vi "Configure Digital Gen Multitone.vi"(6 "Enable Waveform (T: Enable)":bool=TRUE, 7 "Enable EQ Output Modification (T: Enable)":bool=TRUE, 8 "error in (no error)":errorcluster, 9 "Amplitude (0)":dbl, 10 "Channel (0: chA)":i32(ring) items=["chA", "chB"], 11 "VISA resource name":refnum<visa-resource-name>) -> (0 "error out":errorcluster, 3 "VISA resource name out":refnum<visa-resource-name>)   [LabVIEW 2014, in "Stanford Research SR1.lvlib"]
doc: "Configures the attributes for the Digital Generator Multitone.\n\n<b>NOTE</b>: This VI may not be supported by certain models of the SR1."
uses:
  Stanford Research SR1.lvlib
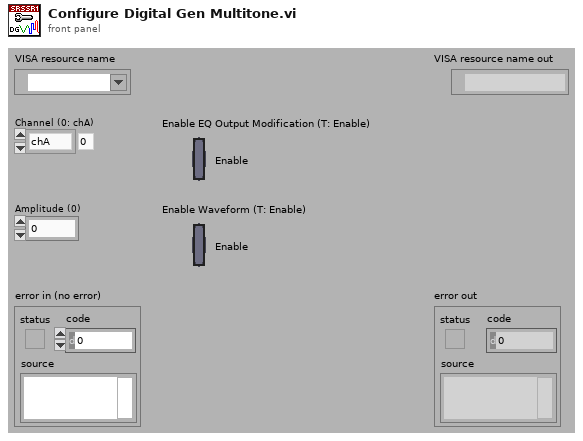
[diagram p1: front panel]
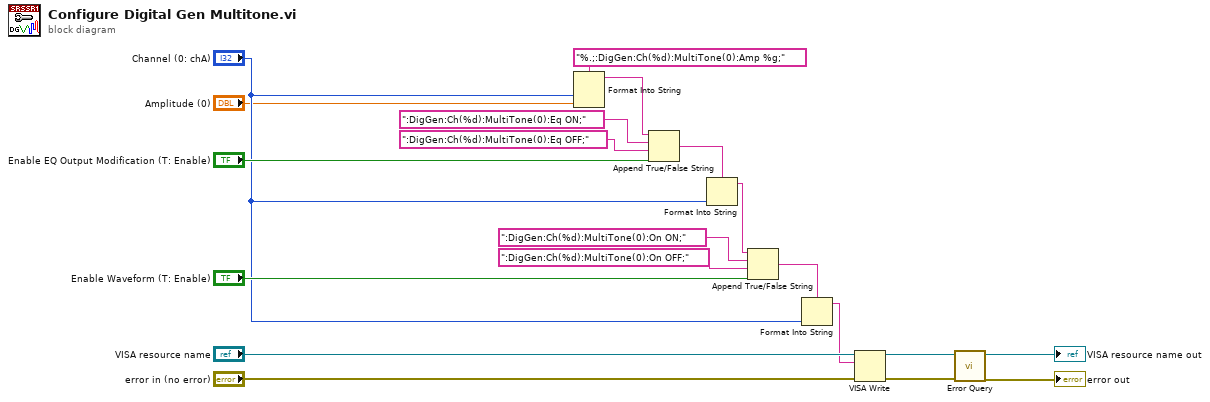
[diagram p0: block diagram]
diagram:
  n1 = Format Into String(format string="%.;:DigGen:Ch(%d):MultiTone(0):Amp %g;", "Channel (0: chA)", "Amplitude (0)") -> (resulting string=w19:string)  [unwired: 2 in, 1 out]
  n2 = Append True/False String(1:"Enable EQ Output Modification (T: Enable)", 2:":DigGen:Ch(%d):MultiTone(0):Eq OFF;", 3:":DigGen:Ch(%d):MultiTone(0):Eq ON;", 4:w19) -> (0:w6:string)
  n3 = Format Into String(format string=w6, "Channel (0: chA)") -> (resulting string=w5:string)  [unwired: 2 in, 1 out]
  n4 = Append True/False String(1:"Enable Waveform (T: Enable)", 2:":DigGen:Ch(%d):MultiTone(0):On OFF;", 3:":DigGen:Ch(%d):MultiTone(0):On ON;", 4:w5) -> (0:w4:string)
  n5 = Format Into String(format string=w4, "Channel (0: chA)") -> (resulting string=w3:string)  [unwired: 2 in, 1 out]
  n6 = VISA Write(VISA resource name="VISA resource name", write buffer=w3, error in (no error)="error in (no error)") -> (VISA resource name out=w10:refnum<visa-resource-name>, error out=w9:errorcluster)  [unwired: 1 out]
  n7 = call "Error Query.vi"("error in (no error)"=w9, "VISA resource name"=w10) -> ("error out"=→"error out":errorcluster, "VISA resource name out"=→"VISA resource name out":refnum<visa-resource-name>)  [unwired: 6 in, 2 out]
